vi "addSetForceFrame.vi"(8 "error in (no error)":errorcluster, 9 "SlewFlag":bool, 10 "ModbusBuffer in":refnum<class "ModbusBuffer.lvclass">, 11 "FAILC in":refnum<class "FAILC.lvclass">) -> (0 "error out":errorcluster, 2 "ModbusBuffer out":refnum<class "ModbusBuffer.lvclass">, 3 "FAILC out":refnum<class "FAILC.lvclass">)   [LabVIEW 2016, in "RTFAILC.lvlib" / "FAILC.lvclass"]
uses:
  FAILC.lvclass
  D:/Code/ts_M1M3Support/Common_RT_ILC/ILC/ILC.lvclass
  Common_RT_Modbus/ModbusBuffer/ModbusBuffer.lvclass
  Common_RT_ILC/ILC/ILC.lvclass/ILC.ctl
  FAILC.lvclass/FAILC.ctl
  DataTypes/FATypes.ctl
  Common_RT_Modbus/ModbusBuffer/ModbusBuffer.lvclass/ModbusBuffer.ctl
  Common_RT_Modbus/DataTypes/ExceptionCodes.ctl
  Common_RT_Modbus/ModbusBuffer/writeByteInstruction.vi
  Common_RT_Modbus/ModbusBuffer/calculateCRC.vi
  RTFAILC.lvlib
  Common_RT_ILC/ILC/ILC.lvclass
  Common_RT_Modbus/RTModbus.lvlib
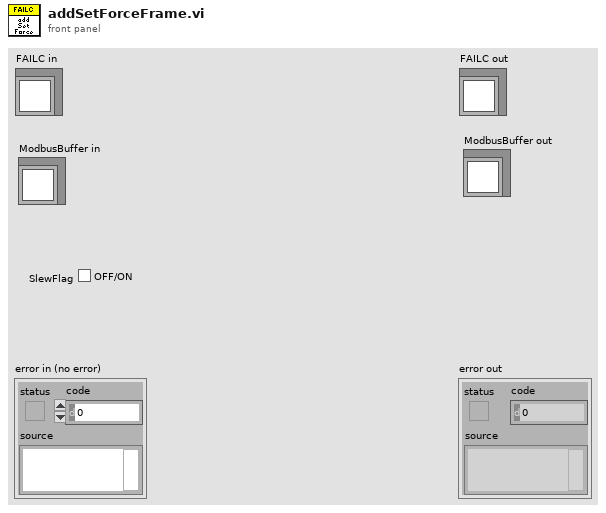
[diagram p1: front panel]
types:
  T1 = typedef "RTModbus.lvlib/ExceptionCodes.ctl" = u16
  T2 = typedef "RTFAILC.lvlib/FATypes.ctl" = enum16{"SingleAxis", "DualAxis"}
  T3 = typedef "RTILC.lvlib/ILCData.ctl" = cluster{"Constants":T4, "Command":T5, "Telemetry":T7, "Responses":T8, "Timestamps":T9, "Timings":T10}
  T4 = typedef "RTILC.lvlib/ILCConstants.ctl" = cluster{"Subnet":u8, "Address":u8}
  T5 = typedef "RTILC.lvlib/ILCCommand.ctl" = cluster{"Mode":u16, "TemporaryAddress":u8, "ADCScanRate":T6, "ADCChannel":u8, "ADCOffset":sgl, "ADCSensitivity":sgl}
  T6 = typedef "RTILC.lvlib/ILCScanRates.ctl" = u8
  T7 = typedef "RTILC.lvlib/ILCTelemetry.ctl" = cluster{"UniqueID":u64, "FirmwareType":u8, "NetworkNodeType":u8, "ILCOption":u8, "NetworkNodeOption":u8, "MajorRevision":u8, "MinorRevision":u8, "FirmwareName":string, "Mode":u16, "MajorFault":bool, "MinorFault":bool, "FaultOverride":bool, "MainCalibrationError":bool, "BackupCalibrationError":bool, "UniqueIDCRCMismatch":bool, "AppTypeNodeTypeMismatch":bool, "AppMissing":bool, "AppCRCMismatch":bool, "TEDSNotFound":bool, "TEDS1Mismatch":bool, "TEDS2Mismatch":bool, "WatchdogResetDetected":bool, "BrownoutDetected":bool, "EventTrapResetDetected":bool, "MotorPowerFault":bool, "SSRPowerFault":bool, "AuxPowerFault":bool, "SMCPowerFault":bool, "TemporaryAddress":u8, "ADCScanRate":T6, "MainADCCalibrationK":sgl[], "MainSensorOffset":sgl[], "MainSensorSensitivity":sgl[], "BackupADCCalibrationK":sgl[], "BackupSensorOffset":sgl[], "BackupSensorSensitivity":sgl[]}
  T8 = typedef "RTILC.lvlib/ILCResponses.ctl" = cluster{"ReportServerID":T1, "ReportServerStatus":T1, "Mode":T1, "TemporaryAddress":T1, "Reset":T1, "ADCScanRate":T1, "ADCOffsetSensitivity":T1, "ReportCalibrationData":T1}
  T9 = typedef "RTILC.lvlib/ILCTimestamps.ctl" = cluster{"ReportServerID":dbl, "ReportServerStatus":dbl, "Mode":dbl, "TemporaryAddress":dbl, "Reset":dbl, "ADCScanRate":dbl, "ADCOffsetSensitivity":dbl, "ReportCalibrationData":dbl}
  T10 = typedef "RTILC.lvlib/ILCTimings.ctl" = cluster{"ReportServerID":u32, "ReportServerStatus":u32, "Mode":u32, "TemporaryAddress":u32, "Reset":u32, "ADCScanRate":u32, "ADCOffsetSensitivity":u32, "ReportCalibrationData":u32}
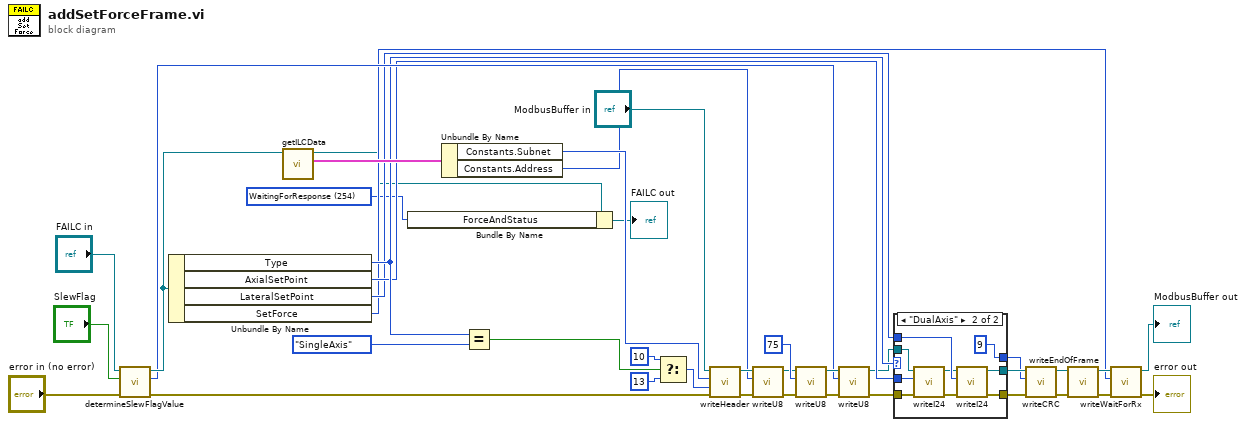
[diagram p0: block diagram]
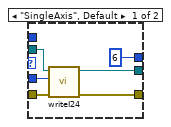
[diagram p2: hidden frame]
diagram:
  w2 = T1 254 items=["OK"=0, "IllegalFunction"=1, "IllegalDataAddress"=2, "IllegalDataValue"=3, "SlaveDeviceFailure"=4, "Acknowledge"=5, "SlaveDeviceBusy"=6, "NegativeAcknowledge"=7, "MemoryParityError"=8, "GatewayPathUnavailable"=9, "GatewayTargetDeviceFailedToRespond"=10, "WaitingForResponse"=254, "CRCError"=255] ("FAData.Responses.ForceAndStatus")
  n1 = call "determineSlewFlagValue.vi"("error in (no error)"="error in (no error)", "SlewFlag"="SlewFlag", "FAILC in"="FAILC in") -> ("error out"=w6:errorcluster, "FlagValue"=w19:u8, "FAILC out"=w20:refnum<class "FAILC.lvclass">)  [unwired: 6 in]
  n2 = Unbundle By Name(w20) -> ("Type"=w16:T2, "AxialSetPoint"=w15:i32, "LateralSetPoint"=w14:i32, "SetForce"=w9:u32)
  n3 = call "getILCData.vi"("ILC in"=w20) -> ("ILCData"=w27:T3, "ILC out"=w3:refnum<class "FAILC.lvclass">)  [unwired: 9 in]
  n4 = Bundle By Name(cluster=w3, "ForceAndStatus"=w2) -> (→"FAILC out":refnum<class "FAILC.lvclass">)
  n5 = Unbundle By Name(w27) -> ("Constants.Subnet"=w26:u8, "Constants.Address"=w25:u8)
  n6 = Equal?(x=w16, y=FATypes."SingleAxis") -> (x = y?=w31:bool)
  n7 = Select(t=u16 10 ("Length"), s=w31, f=u16 13) -> (s? t:f=w28:u16)
  n8 = call "writeHeader.vi"("error in (no error)"=w6, "Length"=w28, "Subnet"=w26, "ModbusBuffer in"="ModbusBuffer in") -> ("error out"=w36:errorcluster, "ModbusBuffer out"=w39:refnum<class "ModbusBuffer.lvclass">)  [unwired: 6 in]
  n9 = call "writeU8.vi"("error in (no error)"=w36, "Input"=w25, "ModbusBuffer in"=w39) -> ("error out"=w35:errorcluster, "ModbusBuffer out"=w24:refnum<class "ModbusBuffer.lvclass">)  [unwired: 7 in]
  n10 = call "writeU8.vi"("error in (no error)"=w35, "Input"=u8 75 ("Function"), "ModbusBuffer in"=w24) -> ("error out"=w18:errorcluster, "ModbusBuffer out"=w23:refnum<class "ModbusBuffer.lvclass">)  [unwired: 7 in]
  n11 = call "writeU8.vi"("error in (no error)"=w18, "Input"=w19, "ModbusBuffer in"=w23) -> ("error out"=w17:errorcluster, "ModbusBuffer out"=w13:refnum<class "ModbusBuffer.lvclass">)  [unwired: 7 in]
  n12 = case shown="\"DualAxis\"" w16 {
    tunnel: w17 -> [w46 w55]
    tunnel: w15 -> [w45 w53]
    tunnel: w14 -> [_ w52]
    tunnel: w13 -> [w42 w50]
    tunnel: [w43 w49] -> w12
    tunnel: [w44 w48] -> w11
    tunnel: [6 ("Length") 9 ("Length")] -> w10
    frame "SingleAxis", Default {
      n13 = call "writeI24.vi"("error in (no error)"=w46, "Input"=w45, "ModbusBuffer in"=w42) -> ("error out"=w44:errorcluster, "ModbusBuffer out"=w43:refnum<class "ModbusBuffer.lvclass">)  [unwired: 7 in]
    }
    frame "DualAxis" {
      n14 = call "writeI24.vi"("error in (no error)"=w55, "Input"=w53, "ModbusBuffer in"=w50) -> ("error out"=w54:errorcluster, "ModbusBuffer out"=w51:refnum<class "ModbusBuffer.lvclass">)  [unwired: 7 in]
      n15 = call "writeI24.vi"("error in (no error)"=w54, "Input"=w52, "ModbusBuffer in"=w51) -> ("error out"=w48:errorcluster, "ModbusBuffer out"=w49:refnum<class "ModbusBuffer.lvclass">)  [unwired: 7 in]
    }
  }
  n16 = call "writeCRC.vi"("error in (no error)"=w11, "Length"=w10, "ModbusBuffer in"=w12) -> ("error out"=w34:errorcluster, "ModbusBuffer out"=w38:refnum<class "ModbusBuffer.lvclass">)  [unwired: 7 in]
  n17 = call "writeEndOfFrame.vi"("error in (no error)"=w34, "ModbusBuffer in"=w38) -> ("error out"=w33:errorcluster, "ModbusBuffer out"=w37:refnum<class "ModbusBuffer.lvclass">)  [unwired: 8 in]
  n18 = call "writeWaitForRx.vi"("error in (no error)"=w33, "Timeout(us)"=w9, "ModbusBuffer in"=w37) -> ("error out"=→"error out":errorcluster, "ModbusBuffer out"=→"ModbusBuffer out":refnum<class "ModbusBuffer.lvclass">)  [unwired: 7 in]
